vi "SubnetOne.vi"() -> (3 "MockFAILCSettings out":refnum<class "MockFAILCSettings.lvclass">)   [LabVIEW 2016, in "FPGAMockFAILC.lvlib"]
uses:
  FPGAMockFAILC.lvlib
  DataTypes/MockFAILCSettings.ctl
  MockFAILCSettings.lvclass
panel:
  in  "MockFAILCSettings class":refnum<class "MockFAILCSettings.lvclass">
  in  "MockFAILCSettings":T1={"ModbusTxDataFIFO"="MockbusPort2TxFIFO", "Code17Memory"="MockFAILC1Code17", "BufferUpdateFIFO"="MockFAILC1Command", "ModbusRxDataFIFO"="MockbusPort2RxFIFO", "Code18Memory"="MockFAILC1Code18", "Code65Memory"="MockFAILC1Code65", "Code66Memory"="MockFAILC1Code66", "Code67Memory"="MockFAILC1Code67", "Code72Memory"="MockFAILC1Code72", "Code80Memory"="MockFAILC1Code80", "Code110Memory"="MockFAILC1Code110", "CRCDataFIFO"="MockFAILC1CRCDataFIFO", "CRCCalculateFIFO"="MockFAILC1CRCCalculateFIFO", "CRCFIFO"="MockFAILC1CRCFIFO"}
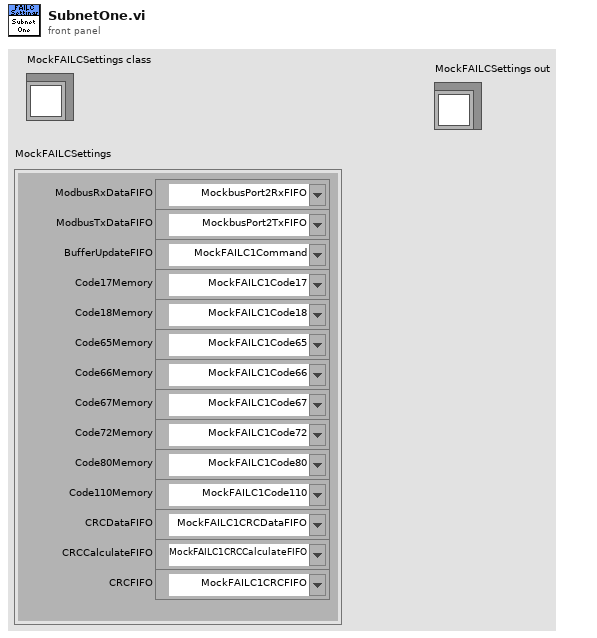
[diagram p1: front panel]
types:
  T1 = typedef "FPGAMockFAILC.lvlib/MockFAILCSettings.ctl" = cluster{"ModbusTxDataFIFO":refnum<k21>, "Code17Memory":refnum<k21>, "BufferUpdateFIFO":refnum<k21>, "ModbusRxDataFIFO":refnum<k21>, "Code18Memory":refnum<k21>, "Code65Memory":refnum<k21>, "Code66Memory":refnum<k21>, "Code67Memory":refnum<k21>, "Code72Memory":refnum<k21>, "Code80Memory":refnum<k21>, "Code110Memory":refnum<k21>, "CRCDataFIFO":refnum<k21>, "CRCCalculateFIFO":refnum<k21>, "CRCFIFO":refnum<k21>}
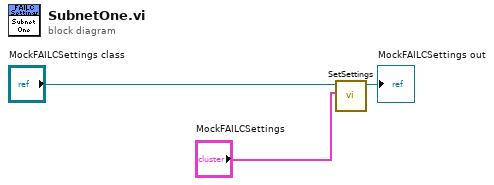
[diagram p0: block diagram]
diagram:
  n1 = call "SetSettings.vi"("MockFAILCSettings"="MockFAILCSettings", "MockFAILCSettings in"="MockFAILCSettings class") -> ("MockFAILCSettings out"=→"MockFAILCSettings out":refnum<class "MockFAILCSettings.lvclass">)  [unwired: 8 in, 1 out]
